vi "Load Step.vi"(8 "error in (no error)":errorcluster, 11 "Step Type":T1) -> (0 "error out":errorcluster, 3 "Step":refnum<class "Step.lvclass">)   [LabVIEW 2020, in "MacroAssert.lvlib"]
doc: "Instantiates a class-based <B>Step</B> object from disk based on <B>Step Type</B>."
uses:
  MacroAssert.lvlib
  CTLs/Step Type v1.ctl
  Step/Step.lvclass
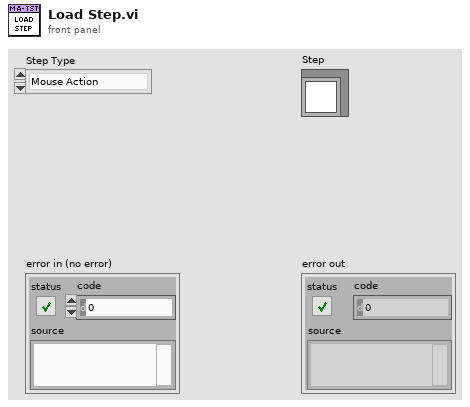
[diagram p1: front panel]
types:
  T1 = typedef "MacroAssert.lvlib/Step Type v1.ctl" = enum16{"Mouse Action", "Keyboard Action", "Window Action", "Timing Action", "Boolean Assertion", "Numeric Assertion", "String Assertion", "Image Assertion"}
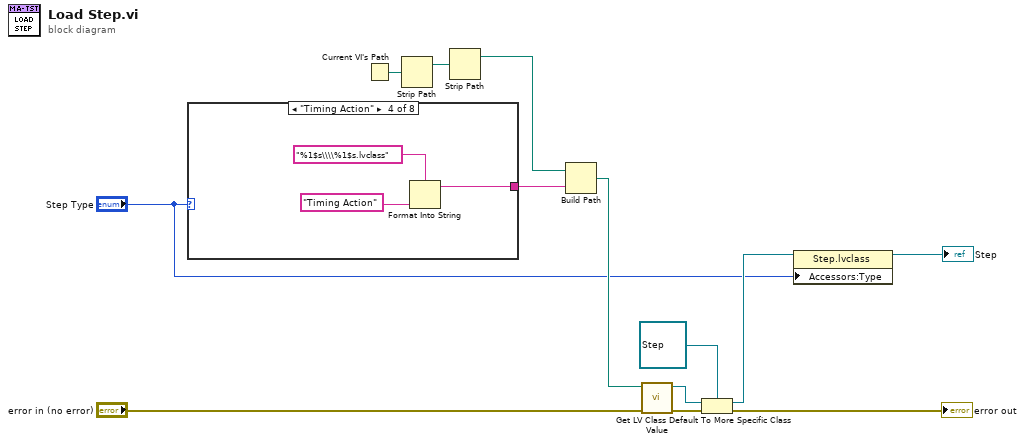
[diagram p0: block diagram]
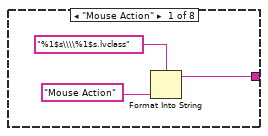
[diagram p2: hidden frame]
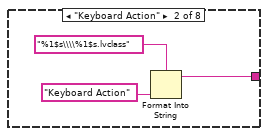
[diagram p3: hidden frame]
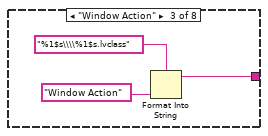
[diagram p4: hidden frame]
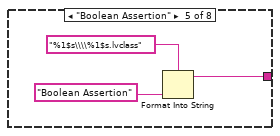
[diagram p5: hidden frame]
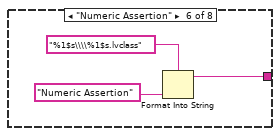
[diagram p6: hidden frame]
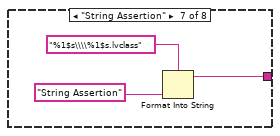
[diagram p7: hidden frame]
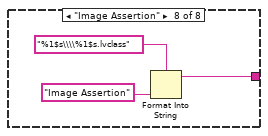
[diagram p8: hidden frame]
diagram:
  n1 = case shown="\"Timing Action\"" "Step Type" {
    tunnel: [w15 w18 w21 w24 w27 w30 w33 w36] -> w5
    frame "Mouse Action" {
      n2 = Format Into String(format string="%1$s\\\\%1$s.lvclass", "Mouse Action") -> (resulting string=w15:string)  [unwired: 2 in, 1 out]
    }
    frame "Keyboard Action" {
      n3 = Format Into String(format string="%1$s\\\\%1$s.lvclass", "Keyboard Action") -> (resulting string=w18:string)  [unwired: 2 in, 1 out]
    }
    frame "Window Action" {
      n4 = Format Into String(format string="%1$s\\\\%1$s.lvclass", "Window Action") -> (resulting string=w21:string)  [unwired: 2 in, 1 out]
    }
    frame "Timing Action" {
      n5 = Format Into String(format string="%1$s\\\\%1$s.lvclass", "Timing Action") -> (resulting string=w24:string)  [unwired: 2 in, 1 out]
    }
    frame "Boolean Assertion" {
      n6 = Format Into String(format string="%1$s\\\\%1$s.lvclass", "Boolean Assertion") -> (resulting string=w27:string)  [unwired: 2 in, 1 out]
    }
    frame "Numeric Assertion" {
      n7 = Format Into String(format string="%1$s\\\\%1$s.lvclass", "Numeric Assertion") -> (resulting string=w30:string)  [unwired: 2 in, 1 out]
    }
    frame "String Assertion" {
      n8 = Format Into String(format string="%1$s\\\\%1$s.lvclass", "String Assertion") -> (resulting string=w33:string)  [unwired: 2 in, 1 out]
    }
    frame "Image Assertion" {
      n9 = Format Into String(format string="%1$s\\\\%1$s.lvclass", "Image Assertion") -> (resulting string=w36:string)  [unwired: 2 in, 1 out]
    }
  }
  n10 = Current VI's Path() -> (path=w7:path)
  n11 = Strip Path(path=w7) -> (stripped path=w6:path)  [unwired: 1 out]
  n12 = Strip Path(path=w6) -> (stripped path=w4:path)  [unwired: 1 out]
  n13 = Build Path(base path=w4, name or relative path=w5) -> (appended path=w3:path)
  n14 = call <vilib>:"Get LV Class Default Value.vi"("error in (no error)"="error in (no error)", "class path"=w3) -> ("error out"=w13:errorcluster, "object"=w10:refnum<class>)  [unwired: 8 in]
  n15 = To More Specific Class(target class=refnum<class "Step.lvclass"> refnum ("MacroAssert.lvlib:Step.lvclass"), reference=w10, error in=w13) -> (specific class reference=w8:refnum<class "Step.lvclass">, error out=→"error out":errorcluster)
  n16 = property class="Step.lvclass"(reference=w8, "Accessors:Type"="Step Type") -> (reference out=→"Step":refnum<class "Step.lvclass">)  [unwired: 1 in, 1 out]
